vi "Configure Setpoint and Ramp.vi"(0 "VISA resource name":refnum<visa-resource-name>, 5 "Output's Control Loop (1:1)":u16(ring)=1 items=["1"=1, "2"=2], 7 "Setpoint (0.0000)":dbl format="%.4f", 9 "Enable Setpoint Ramping (F: Off)":bool, 11 "error in (no error)":errorcluster, 12 "Ramp Rate (0.0)":dbl format="%.1f") -> (4 "VISA resource name out":refnum<visa-resource-name>, 15 "error out":errorcluster)   [LabVIEW 2012, in "Lake Shore 335.lvlib"]
doc: "Configures the Setpoint and Setpoint Ramping function. The Setpoint parameter is used to set the desired load temperature for a control loop."
uses:
  <instrlib>/lake shore 335/Temperature control panel Folder/C/Program Files/National Instruments/LabVIEW 2013/instr.lib/lake shore 335/Lake Shore 335.lvlib
  Instance           1 35Saved   Configure Setpoint and Ramp .vi
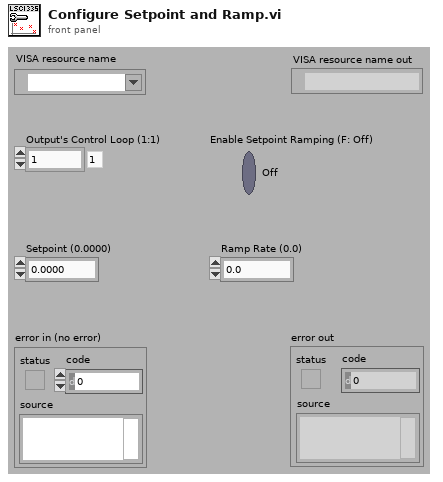
[diagram p1: front panel]
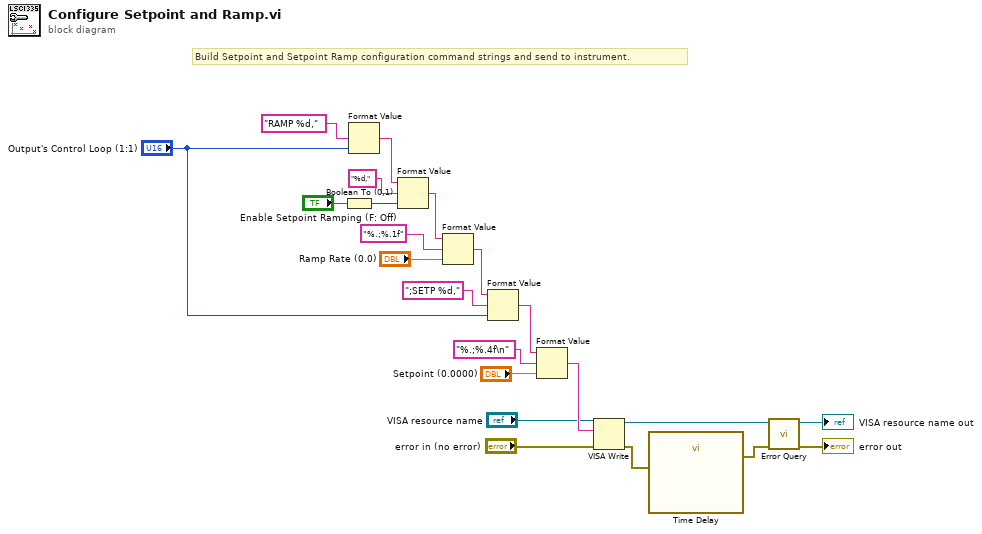
[diagram p0: block diagram]
diagram:
  # "Build Setpoint and Setpoint Ramp configuration command strings and send to instrument."
  n1 = Boolean To (0,1)(Boolean="Enable Setpoint Ramping (F: Off)") -> (0, 1=w6:i16)
  n2 = Format Value(format string="RAMP %d,", value (0)="Output's Control Loop (1:1)") -> (output string=w12:string)  [unwired: 1 in]
  n3 = Format Value(string ("")=w12, format string="%d,", value (0)=w6) -> (output string=w8:string)
  n4 = Format Value(string ("")=w8, format string="%.;%.1f", value (0)="Ramp Rate (0.0)") -> (output string=w4:string)
  n5 = Format Value(string ("")=w4, format string=";SETP %d,", value (0)="Output's Control Loop (1:1)") -> (output string=w13:string)
  n6 = Format Value(string ("")=w13, format string="%.;%.4f\n", value (0)="Setpoint (0.0000)") -> (output string=w15:string)
  n7 = VISA Write(VISA resource name="VISA resource name", write buffer=w15, error in (no error)="error in (no error)") -> (VISA resource name out=w22:refnum<visa-resource-name>, error out=w19:errorcluster)  [unwired: 1 out]
  n8 = call "Time Delay"("error in (no error)"=w19) -> ("error out"=w18:errorcluster)  [unwired: 10 in]
  n9 = call <instrlib>:"Error Query.vi"("error in (no error)"=w18, "VISA resource name"=w22) -> ("error out"=→"error out":errorcluster, "VISA resource name out"=→"VISA resource name out":refnum<visa-resource-name>)  [unwired: 7 in, 1 out]
